vi "WRAPPER Start Log and Sequence.vi"(8 "error in (no error)":errorcluster, 11 "Stim Player Data In":T2) -> (0 "error out":errorcluster, 2 "SessComplEvent":T1, 3 "Stim Player Data Out":T2)   [LabVIEW 2011]
uses:
  Controls/Stim Player Data.ctl
  Controls/Top Level Control.ctl
  <vilib>/NI/AMC/Message Queue.ctl
  <vilib>/NI/AMC/Message.ctl
  <vilib>/NI/Tools/Keyed Array/KeyedArray.ctl
  Controls/ListBox Test Record.ctl
  Controls/DVR of CSV Tests Data.ctl
  Controls/CSVs Tests Data.ctl
  Controls/Test Column Data.ctl
  Controls/Options DVR.ctl
  Controls/Options.ctl
  <vilib>/NI Veristand/Execution/Workspace/WorkspaceAPI.ctl
  NationalInstruments.VeriStand.ClientAPI
  <vilib>/NI Veristand/Execution/SequenceExecutionInterface/Stimulus Profile Session Ref.ctl
  <vilib>/NI Veristand/Execution/ChannelFaultManager/ChannelFaultAPI.ctl
  <vilib>/NI Veristand/Execution/SequenceExecutionInterface/Session Event Ref.ctl
  Sequence Play/Alias or Channel Lookup.vi
  <vilib>/NI Veristand/Execution/SequenceExecutionInterface/Register for Stimulus Profile Session Complete Event.vi
  <vilib>/NI Veristand/Execution/SequenceExecutionInterface/Deploy Stimulus Profile Session.vi
  <vilib>/NI Veristand/Execution/Workspace/NI VeriStand - Start Data Logging.vi
  <vilib>/NI Veristand/Execution/Workspace/NI VeriStand - Get System State.vi
  <vilib>/NI Veristand/Execution/Workspace/NI VeriStand - Get Alias List.vi
  <vilib>/NI Veristand/Execution/Workspace/NI VeriStand - Get System Node Channel List.vi
  <vilib>/NI/Tools/Keyed Array/Tools_KeyedArray.lvlib
  <vilib>/NI/AMC/AMC.lvlib
  <vilib>/NI Veristand/Execution/Workspace/NI_VS Workspace ExecutionAPI.lvlib
  <vilib>/NI Veristand/Execution/SequenceExecutionInterface/NI_VS Sequence Execution Interface.lvlib
  <vilib>/NI Veristand/Execution/ChannelFaultManager/NI_VS ChannelFault ExecutionAPI.lvlib
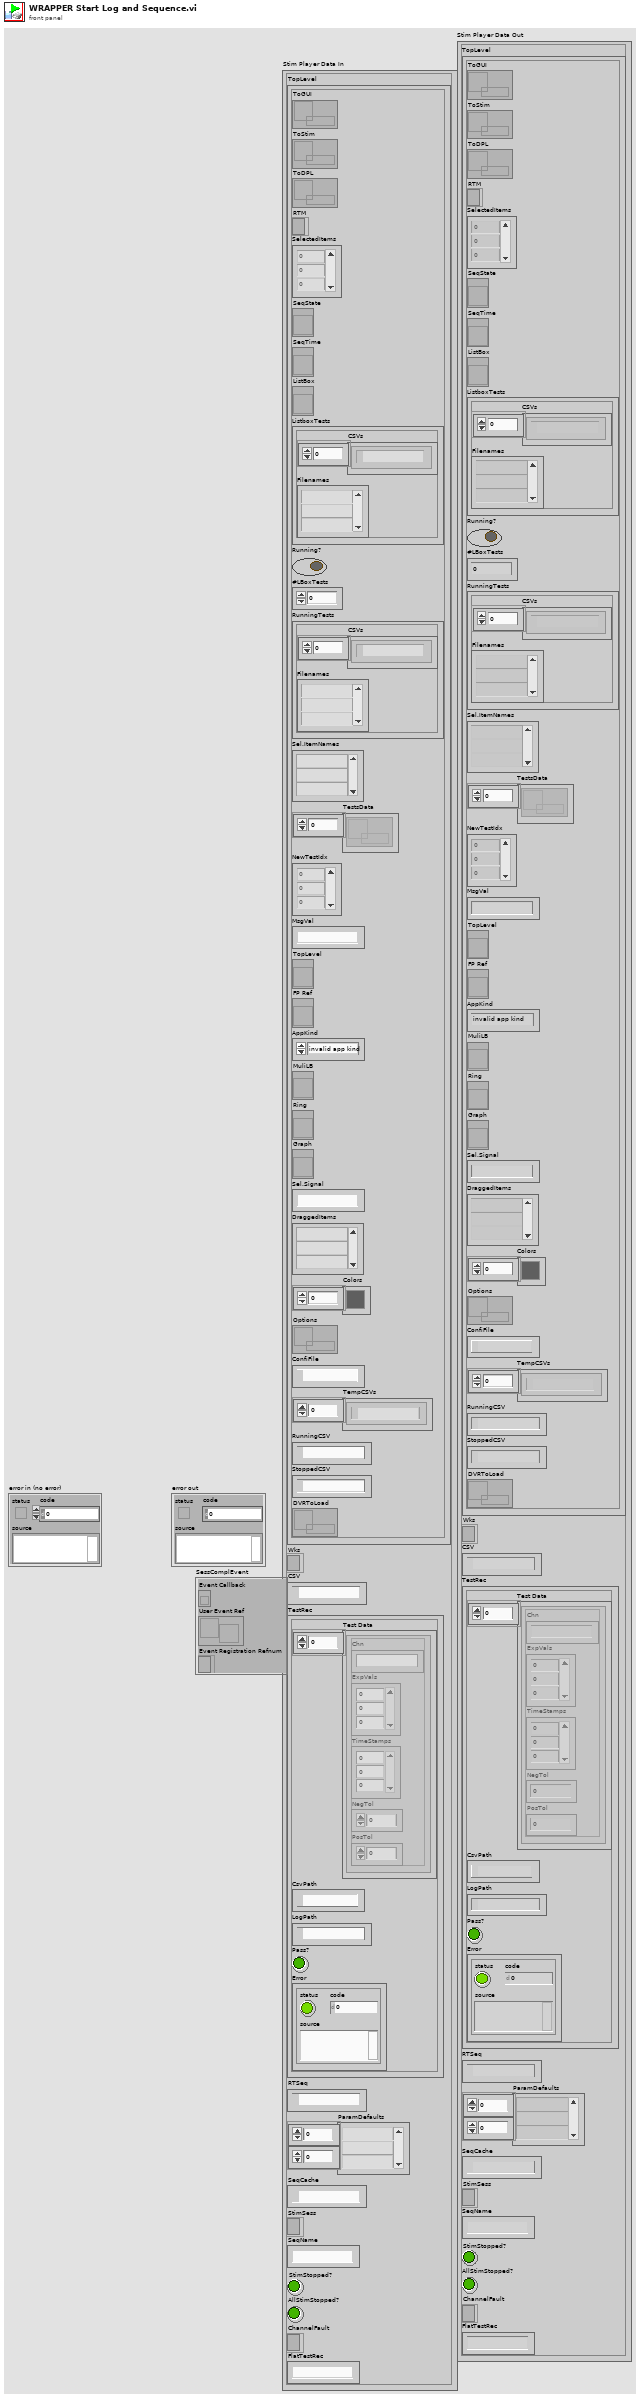
[diagram p1: front panel]
types:
  T1 = typedef "NI_VS Sequence Execution Interface.lvlib/Session Event Ref.ctl" = cluster{"Event Callback":refnum<k27>, "User Event Ref":refnum<user-event>, "Event Registration Refnum":refnum<event-registration>}
  T2 = typedef "Stim Player Data.ctl" = cluster{"TopLevel":T3, "Wks":T8, "CSV":path, "TestRec":T9, "RTSeq":path, "ParamDefaults":string[][], "SeqCache":path, "StimSess":T11, "SeqName":string, "StimStopped?":bool, "AllStimStopped?":bool, "ChannelFault":T12, "FlatTestRec":string}
  T3 = typedef "Top Level Control.ctl" = cluster{"ToGUI":T4, "ToStim":T4, "ToDPL":T4, "RTM":refnum<k9>, "SelectedItems":i32[], "SeqState":refnum<vi>, "SeqTime":refnum<vi>, "ListBox":refnum<vi>, "ListboxTests":T5, "Running?":bool, "#LBoxTests":i32, "RunningTests":T5, "Sel.ItemNames":string[], "TestsData":T6[], "NewTestIdx":i32[], "MsgVal":string, "TopLevel":refnum<vi>, "FP Ref":refnum<vi>, "AppKind":enum32{"invalid app kind", "Development System", "Run Time System", "Student Edition", "Embedded LabVIEW", "Evaluation", "Custom"}, "MuliLB":refnum<vi>, "Ring":refnum<vi>, "Graph":refnum<vi>, "Sel.Signal":string, "DraggedItems":string[], "Colors":u32[], "Options":T7, "ConfiFile":path, "TempCSVs":path[], "RunningCSV":path, "StoppedCSV":path, "DVRToLoad":T6}
  T4 = typedef "AMC.lvlib/Message Queue.ctl" = refnum<queue>
  T5 = typedef "ListBox Test Record.ctl" = cluster{"CSVs":path[], "Filenames":string[]}
  T6 = typedef "DVR of CSV Tests Data.ctl" = refnum<data-value>
  T7 = typedef "Options DVR.ctl" = refnum<data-value>
  T8 = typedef "NI_VS Workspace ExecutionAPI.lvlib/WorkspaceAPI.ctl" = refnum<k24>
  T9 = typedef "CSVs Tests Data.ctl" = cluster{"Test Data":T10[], "CsvPath":path, "LogPath":path, "Pass?":bool, "Error":errorcluster}
  T10 = typedef "Test Column Data.ctl" = cluster{"Chn":string, "ExpVals":dbl[], "TimeStamps":i64[], "NegTol":dbl, "PosTol":dbl}
  T11 = typedef "NI_VS Sequence Execution Interface.lvlib/Stimulus Profile Session Ref.ctl" = refnum<k24>
  T12 = typedef "NI_VS ChannelFault ExecutionAPI.lvlib/ChannelFaultAPI.ctl" = refnum<k24>
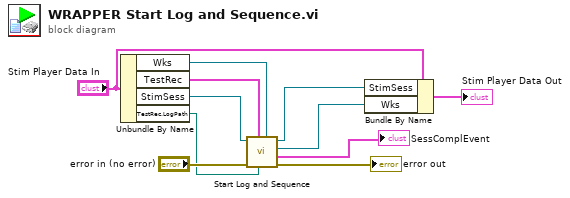
[diagram p0: block diagram]
diagram:
  n1 = Unbundle By Name("Stim Player Data In") -> ("Wks"=w7:T8, "TestRec"=w6:T9, "StimSess"=w5:T11, "TestRec.LogPath"=w4:path)
  n2 = call "Start Log and Sequence.vi"("WorkspaceManager"=w7, "Log File Path"=w4, "Test Columns in"=w6, "error in (no error)"="error in (no error)", "Stim Session"=w5) -> ("error out"=→"error out":errorcluster, "Session Complete Event Ref"=→"SessComplEvent":T1, "WorkspaceManager out"=w2:T8, "Stim Session out"=w3:T11)  [unwired: 3 in]
  n3 = Bundle By Name(cluster="Stim Player Data In", "StimSess"=w3, "Wks"=w2) -> (→"Stim Player Data Out":T2)
